vi "Host.vi"() -> ()   [LabVIEW 2018]
uses:
  <vilib>/userdefined/High Color/nirio_resource_hc.ctl
  <instrlib>/niDCPower/nidcpower.llb/niDCPower Measurement Type.ctl
  <vilib>/FPGAPlugInAG/PXI-7953R/niLvFpga_Open_PXI-7953R.vi
  <vilib>/rvi/interface/common/dynamic/niFpgaDynamicAddResources.vi
  <vilib>/FPGAPlugInAG/Dynamic/niLvFpga_Reset_Dynamic.vi
  <vilib>/FPGAPlugInAG/Dynamic/niLvFpga_Run_Dynamic.vi
  <vilib>/Utility/error.llb/Error Cluster From Error Code.vi
  <vilib>/rvi/errors/niLvFpgaAdjustHostInterfaceError.vi
  <vilib>/FPGAPlugInAG/Dynamic/niLvFpga_Close_Dynamic.vi
  <vilib>/rvi/interface/nirviOpenFPGA/nirviOpenFPGA.xnode
  FPGA Bitfiles/Century22052_FPGATarget_Target_F4PYkC+UQnQ.lvbitx
  <vilib>/rvi/interface/nirviMethod/nirviMethod.xnode
  <vilib>/rvi/interface/nirviReadWriteControl/nirviReadWriteControl.xnode
  <vilib>/rvi/interface/nirviCloseFPGA/nirviCloseFPGA.xnode
  NiFpgaLv.dll
  <vilib>/rvi/interface/Simulation/niFpgaSimulationCallBeginRW.vi
panel:
  in  "Тест №":enum16{"3", "2", "1"}(ring)=enum."1"
  in  "Сообщение":bool
  in  "RESET":bool=TRUE
  in  "A0":bool
  in  "SEL_T, мс":u32=100
  in  "SIM_SEL":bool
  out "SEL":bool
  in  "VCC_selcur":dbl=0.89 caption="current limit" format="%_6p"
  out "VCC":i32
  out "VCC":bool
  in  "Период опроса, мс":u32=1000
  in  "VCC, V":dbl=5.0 caption="voltage level" format="%_6p"
  in  "VCC_curlim, A":dbl=1.0 caption="current limit" format="%_6p"
  in  "6581_curlim, A":dbl=1.0 caption="current limit" format="%_6p"
  out "VCC_cur, A":dbl caption="measurement" format="%_6g"
  out "6581_cur, A":dbl caption="measurement" format="%_6g"
  in  "6581, V":dbl=5.0 caption="voltage level" format="%_6p"
  out "6581 Chart":dbl(graph)=0.0006520018718277456
  out "VCC Chart":dbl(graph)=0.09491557293549348 caption="Waveform Chart 5"
  in  "Стоп":bool
  in  "Питание":bool
  in  "VСС_6581_5V":refnum<k15>="PXI1Slot2" caption="instrument handle"
  in  "resource name":T1="PXI1Slot6"
  in  "SEL":path=path "C:/VPL/LabView_PRJ/Century_22052/SEL"
  out "Номер образца":string="0"
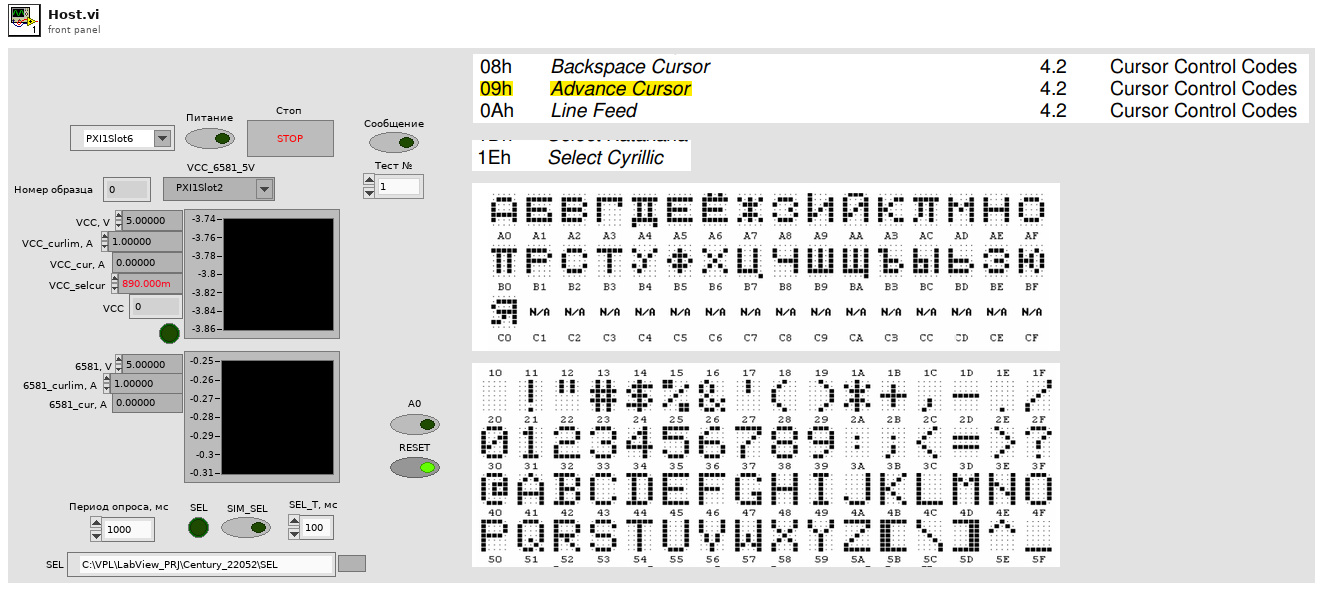
[diagram p1: front panel]
types:
  T1 = typedef "nirio_resource_hc.ctl" = tag
  T2 = enum16{"open", "replace", "create", "open or create", "replace or create", "replace or create with confirmation"}
  T3 = typedef "niDCPower Measurement Type.ctl" = i32
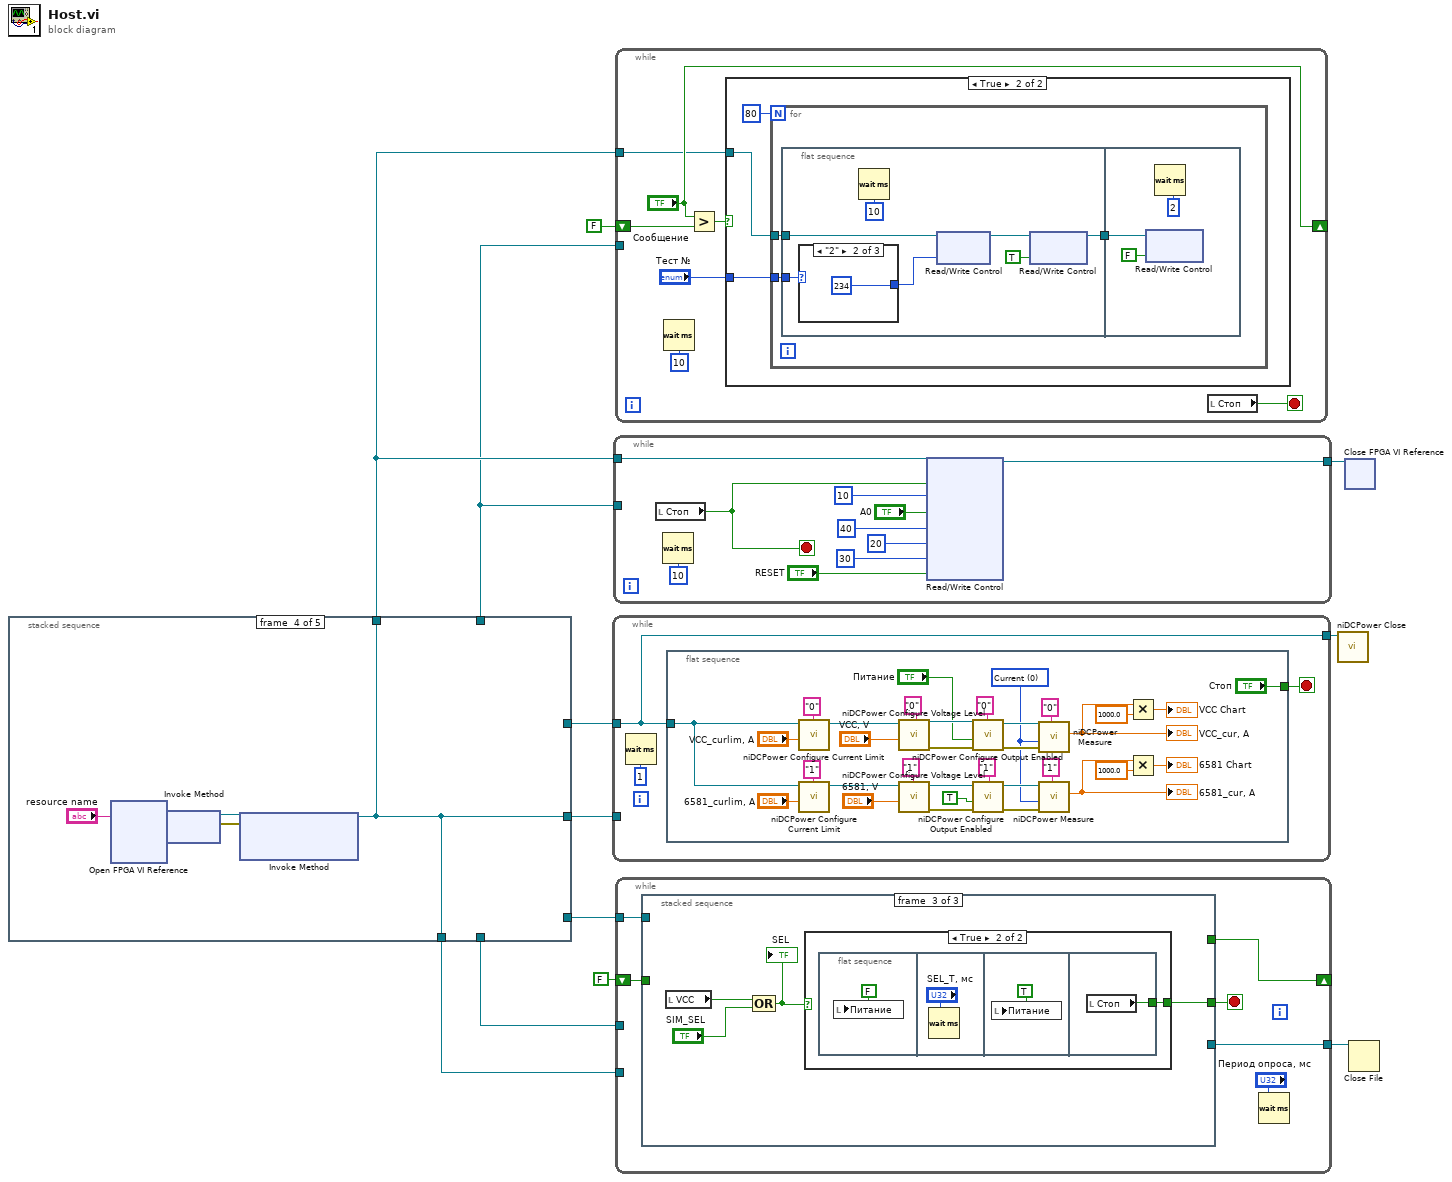
[diagram p0: block diagram]
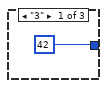
[diagram p3: hidden frame]
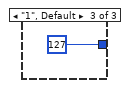
[diagram p4: hidden frame]
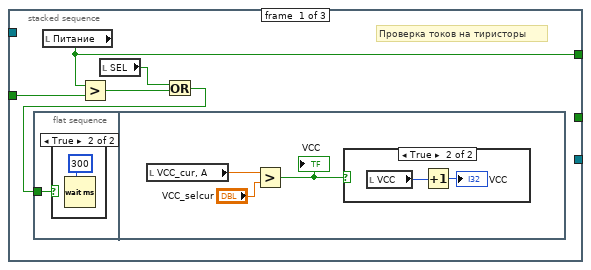
[diagram p5: hidden frame]
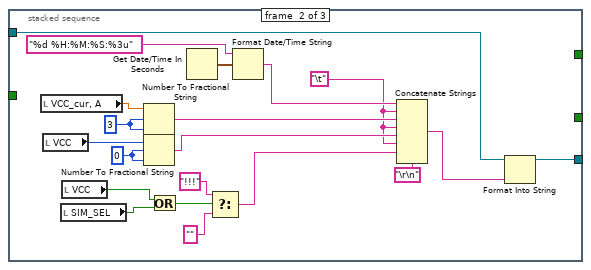
[diagram p8: hidden frame]
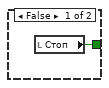
[diagram p9: hidden frame]
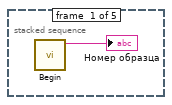
[diagram p10: hidden frame]
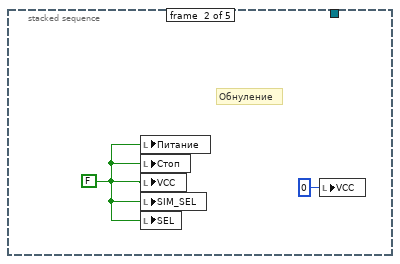
[diagram p11: hidden frame]
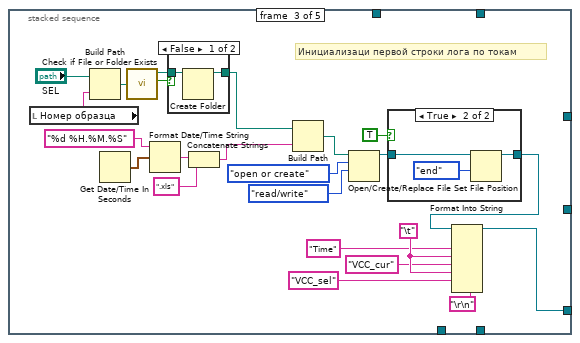
[diagram p12: hidden frame]
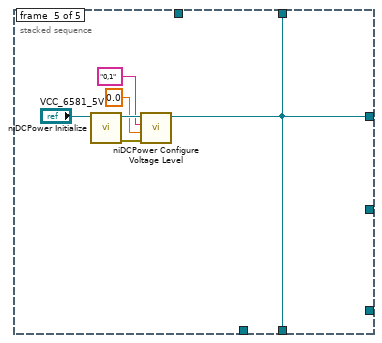
[diagram p15: hidden frame]
diagram:
  n1 = stacked-sequence {
    tunnel: [_ _ _ w46 _] -> w6
    tunnel: [_ _ w21 _ _] -> w7
    tunnel: [_ _ _ w46 _] -> w5
    tunnel: [_ _ _ w46 _] -> w3
    tunnel: [_ _ _ _ w52] -> w9
    tunnel: [_ _ _ _ w52] -> w8
    tunnel: [_ _ _ _ w52] -> w2
    frame #0 {
      n2 = call "Begin.vi"() -> ("Номер образца 2"=→"Номер образца":string)  [unwired: 11 in]
    }
    frame #1 {
      w15 = FALSE
      # "Обнуление"
      n3 = local write "Питание"(w15) -> ()
      n4 = local write "Стоп"(w15) -> ()
      n5 = local write "VCC"(w15) -> ()
      n6 = local write "SIM_SEL"(w15) -> ()
      n7 = local write "SEL"(w15) -> ()
      n8 = local write "VCC"(0 ("VCC")) -> ()
    }
    frame #2 {
      w22 = "\t"
      # "Инициализаци первой строки лога по токам"
      n9 = local read "Номер образца"() -> (w34:string)
      n10 = Build Path(base path="SEL", name or relative path=w34) -> (appended path=w36:path)
      n11 = Get Date/Time In Seconds() -> (seconds since 1Jan1904=w29:timestamp)
      n12 = call <vilib>:"Check if File or Folder Exists.vi"("path"=w36) -> ("file or folder exists?"=w37:bool, "dup path"=w38:path)  [unwired: 8 in, 1 out]
      n13 = Format Date/Time String(time format string (%c)="%d %H.%M.%S", seconds (now)=w29) -> (date/time string=w26:string)  [unwired: 1 in]
      n14 = case shown="False" w37 {
        tunnel: w38 -> [w44 w45]
        tunnel: [w43 w45] -> w20
        frame False {
          n15 = Create Folder(path (use dialog)=w44) -> (created path=w43:path)  [unwired: 2 in, 2 out]
        }
        frame True {
        }
      }
      n16 = Concatenate Strings(w26, ".xls" ("string")) -> (w24:string)
      n17 = Build Path(base path=w20, name or relative path=w24) -> (appended path=w27:path)
      n18 = Open/Create/Replace File(file path (use dialog)=w27, operation (0:open)=T2."open or create", access (0:read/write)=enum16{"read/write", "read-only", "write-only"}."read/write") -> (refnum out=w30:refnum<file>)  [unwired: 3 in, 2 out]
      n19 = case shown="True" TRUE {
        tunnel: w30 -> [w39 w42]
        tunnel: [w39 w40] -> w23
        frame False {
        }
        frame True {
          n20 = Set File Position(refnum=w42, from (0:start)=enum16{"start", "end", "current"}."end") -> (refnum out=w40:refnum<file>)  [unwired: 2 in, 1 out]
        }
      }
      n21 = Format Into String(initial string=w23, "Time" ("input 1"), w22, "VСС_cur" ("input 1"), w22, "VСС_sel" ("input 1"), "\r\n") -> (resulting string=w21:refnum<file>)  [unwired: 2 in, 1 out]
    }
    frame #3 {
      n22 = xnode "Open FPGA VI Reference"("resource name"="resource name") -> ("FPGA VI Reference Out"=w51:refnum<k20>, "error out"=w49:errorcluster)  [unwired: 1 in]
      n23 = xnode "Invoke Method"("FPGA VI Reference In"=w51, "error in"=w49) -> ("FPGA VI Reference Out"=w48:refnum<k20>, "error out"=w50:errorcluster)
      n24 = xnode "Invoke Method"("FPGA VI Reference In"=w48, "error in"=w50) -> ("FPGA VI Reference Out"=w46:refnum<k20>)  [unwired: 1 in, 1 out]
    }
    frame #4 {
      n25 = call <instrlib>:"niDCPower Initialize.vi"("resource name"="VСС_6581_5V") -> ("error out"=w56:errorcluster, "instrument handle out"=w57:refnum<k15>)  [unwired: 3 in, 6 out]
      n26 = call <instrlib>:"niDCPower Configure Voltage Level.vi"("error in (no error)"=w56, "voltage level"=0.0, "channel name"="0,1", "instrument handle"=w57) -> ("instrument handle out"=w52:refnum<k15>)  [unwired: 6 in, 1 out]
    }
  }
  n27 = while {
    tunnel: w9 -> [w58]
    tunnel: [w58] -> w10
    tunnel: w6 -> [_]
    stop <- w59 stop-if-true
    n28 = Wait (ms)(milliseconds to wait=u32 1) -> ()  [unwired: 1 out]
    n29 = flat-sequence {
      tunnel: w58 -> [w66]
      tunnel: ["Стоп"] -> w59
      frame #0 {
        w62 = T3 0 items=["Current", "Voltage"] ("measurement type")
        n30 = call <instrlib>:"niDCPower Configure Current Limit.vi"("current limit"="VCC_curlim, A", "channel name"="0", "instrument handle"=w66) -> ("instrument handle out"=w83:refnum<k15>)  [unwired: 7 in, 1 out]
        n31 = call <instrlib>:"niDCPower Configure Current Limit.vi"("current limit"="6581_curlim, A", "channel name"="1", "instrument handle"=w66) -> ("instrument handle out"=w84:refnum<k15>)  [unwired: 7 in, 1 out]
        n32 = call <instrlib>:"niDCPower Configure Voltage Level.vi"("voltage level"="VCC, V", "channel name"="0", "instrument handle"=w83) -> ("error out"=w76:errorcluster, "instrument handle out"=w79:refnum<k15>)  [unwired: 7 in]
        n33 = call <instrlib>:"niDCPower Configure Voltage Level.vi"("voltage level"="6581, V", "channel name"="1", "instrument handle"=w84) -> ("error out"=w77:errorcluster, "instrument handle out"=w78:refnum<k15>)  [unwired: 7 in]
        n34 = call <instrlib>:"niDCPower Configure Output Enabled.vi"("error in (no error)"=w76, "output enabled"="Питание", "channel name"="0", "instrument handle"=w79) -> ("error out"=w88:errorcluster, "instrument handle out"=w87:refnum<k15>)  [unwired: 6 in]
        n35 = call <instrlib>:"niDCPower Configure Output Enabled.vi"("error in (no error)"=w77, "output enabled"=TRUE, "channel name"="1", "instrument handle"=w78) -> ("error out"=w89:errorcluster, "instrument handle out"=w90:refnum<k15>)  [unwired: 6 in]
        n36 = call <instrlib>:"niDCPower Measure.vi"("error in (no error)"=w88, "measurement type"=w62, "channel name"="0", "instrument handle"=w87) -> ("measurement"=w69:dbl)  [unwired: 5 in, 2 out]
        "VCC_cur, A" <- w69
        n37 = call <instrlib>:"niDCPower Measure.vi"("error in (no error)"=w89, "measurement type"=w62, "channel name"="1", "instrument handle"=w90) -> ("measurement"=w70:dbl)  [unwired: 5 in, 2 out]
        "6581_cur, A" <- w70
        n38 = Multiply(x=w69, y=1000.0) -> (x*y=→"VCC Chart":dbl)
        n39 = Multiply(x=w70, y=1000.0) -> (x*y=→"6581 Chart":dbl)
      }
    }
  }
  n40 = while {
    tunnel: w3 -> [w102]
    tunnel: w2 -> [_]
    tunnel: [w94] -> w4
    stop <- w101 stop-if-true
    n41 = local read "Стоп"() -> (w101:bool)
    n42 = Wait (ms)(milliseconds to wait=u32 10) -> ()  [unwired: 1 out]
    n43 = xnode "Read/Write Control"("FPGA VI Reference In"=w102, "Stop_FPGA"=w101, "10"=10, "A0"="A0", "40"=40, "20"=20, "30"=30, "RESET"="RESET") -> ("FPGA VI Reference Out"=w94:refnum<k20>)  [unwired: 1 in, 1 out]
  }
  n44 = while {
    tunnel: w3 -> [w105]
    tunnel: w2 -> [_]
    shift-right: ["Сообщение"] -> _
    shift-left: FALSE ("Сообщение") -> [w110]
    stop <- w108 stop-if-true
    n45 = Wait (ms)(milliseconds to wait=u32 10) -> ()  [unwired: 1 out]
    n46 = Greater?(x="Сообщение", y=w110) -> (0:w107:bool)
    n47 = case shown="True" w107 {
      tunnel: "Тест №" -> [_ w113]
      tunnel: w105 -> [_ w111]
      frame False {
      }
      frame True {
        n48 = for {
          N: 80 -> [_]
          tunnel: w113 -> [w116]
          tunnel: w111 -> [w115]
          n49 = flat-sequence {
            tunnel: w116 -> [w123]
            tunnel: w115 -> [w122]
            tunnel: [w117] -> w114
            tunnel: w114 -> [w129]
            frame #0 {
              n50 = case shown="\"2\"" w123 {
                tunnel: [42 234 127] -> w121
                frame "3" {
                }
                frame "2" {
                }
                frame "1", Default {
                }
              }
              n51 = Wait (ms)(milliseconds to wait=u32 10) -> ()  [unwired: 1 out]
              n52 = xnode "Read/Write Control"("FPGA VI Reference In"=w122, "DATA"=w121) -> ("FPGA VI Reference Out"=w120:refnum<k20>)  [unwired: 1 in, 1 out]
              n53 = xnode "Read/Write Control"("FPGA VI Reference In"=w120, "Запись"=TRUE) -> ("FPGA VI Reference Out"=w117:refnum<k20>)  [unwired: 1 in, 1 out]
            }
            frame #1 {
              n54 = xnode "Read/Write Control"("FPGA VI Reference In"=w129, "Запись"=FALSE) -> ()  [unwired: 1 in, 2 out]
              n55 = Wait (ms)(milliseconds to wait=u32 2) -> ()  [unwired: 1 out]
            }
          }
        }
      }
    }
    n56 = local read "Стоп"() -> (w108:bool)
  }
  n57 = while {
    shift-right: [w135] -> _
    shift-left: FALSE -> [w134]
    tunnel: w7 -> [w133]
    tunnel: [w131] -> w11
    tunnel: w8 -> [_]
    tunnel: w5 -> [_]
    stop <- w132 stop-if-true
    n58 = stacked-sequence {
      tunnel: [w139 _ _] -> w135
      tunnel: w134 -> [w140 _ _]
      tunnel: w133 -> [_ w160 _]
      tunnel: [_ _ w169] -> w132
      tunnel: [_ w156 _] -> w131
      frame #0 {
        # "Проверка токов на тиристоры"
        n59 = flat-sequence {
          tunnel: w136 -> [w141]
          frame #0 {
            n60 = case shown="True" w141 {
              frame False {
              }
              frame True {
                n61 = Wait (ms)(milliseconds to wait=u32 300) -> ()  [unwired: 1 out]
              }
            }
          }
          frame #1 {
            n62 = local read "VCC_cur, A"() -> (w143:dbl)
            n63 = Greater?(x=w143, y="VCC_selcur") -> (0:w144:bool)
            "VCC" <- w144
            n64 = case shown="True" w144 {
              frame False {
              }
              frame True {
                n65 = local read "VCC"() -> (w147:i32)
                n66 = Increment(x=w147) -> (x+1=→"VCC":i32)
              }
            }
          }
        }
        n67 = local read "Питание"() -> (w139:bool)
        n68 = Greater?(x=w139, y=w140) -> (0:w138:bool)
        n69 = local read "SEL"() -> (w137:bool)
        n70 = Or(x=w137, y=w138) -> (x .or. y?=w136:bool)
      }
      frame #1 {
        w158 = i16 0 ("width (-)")
        w157 = i16 3 ("width (-)")
        w153 = "\t"
        n71 = local read "VCC_cur, A"() -> (w159:dbl)
        n72 = local read "VCC"() -> (w154:i32)
        n73 = local read "SIM_SEL"() -> (w152:bool)
        n74 = local read "VCC"() -> (w151:bool)
        n75 = Number To Fractional String(number=w159, width (-)=w157, precision (6)=w157) -> (F-format string=w161:string)  [unwired: 1 in]
        n76 = Number To Fractional String(number=w154, width (-)=w158, precision (6)=w158) -> (F-format string=w155:string)  [unwired: 1 in]
        n77 = Or(x=w151, y=w152) -> (x .or. y?=w150:bool)
        n78 = Get Date/Time In Seconds() -> (seconds since 1Jan1904=w167:timestamp)
        n79 = Select(t="!!!", s=w150, f="") -> (s? t:f=w149:string)
        n80 = Format Date/Time String(time format string (%c)="%d %H:%M:%S:%3u", seconds (now)=w167) -> (date/time string=w162:string)  [unwired: 1 in]
        n81 = Concatenate Strings(w162, w153, w161, w153, w155, w153, w149, "\r\n") -> (w166:string)
        n82 = Format Into String(initial string=w160, w166) -> (resulting string=w156:refnum<file>)  [unwired: 2 in, 1 out]
      }
      frame #2 {
        n83 = local read "VCC"() -> (w171:bool)
        n84 = Compound Arithmetic op=OR(w171, "SIM_SEL") -> (w170:bool)
        "SEL" <- w170
        n85 = case shown="True" w170 {
          tunnel: [w172 w173] -> w169
          frame False {
            n86 = local read "Стоп"() -> (w172:bool)
          }
          frame True {
            n87 = flat-sequence {
              tunnel: [w177] -> w173
              frame #0 {
                n88 = local write "Питание"(FALSE ("SYS_RESET")) -> ()
              }
              frame #1 {
                n89 = Wait (ms)(milliseconds to wait="SEL_T, мс") -> ()  [unwired: 1 out]
              }
              frame #2 {
                n90 = local write "Питание"(TRUE ("SYS_RESET")) -> ()
              }
              frame #3 {
                n91 = local read "Стоп"() -> (w177:bool)
              }
            }
          }
        }
      }
    }
    n92 = Wait (ms)(milliseconds to wait="Период опроса, мс") -> ()  [unwired: 1 out]
  }
  n93 = call <instrlib>:"niDCPower Close.vi"("instrument handle"=w10) -> ()  [unwired: 10 in, 1 out]
  n94 = xnode "Close FPGA VI Reference"("FPGA VI Reference In"=w4) -> ()  [unwired: 1 in, 1 out]
  n95 = Close File(refnum=w11) -> ()  [unwired: 1 in, 2 out]
